vi "Sub_Conn_Status_FGV.vi"(6 "Connection Status in":T1=enum."Connection refused: not authorized", 8 "error in":errorcluster, 10 "Command":T2) -> (0 "error out":errorcluster, 4 "Connection Status out":T1=enum."Connection refused: not authorized")   [LabVIEW 2019, in "MQTT_Functions.lvlib"]
uses:
  MQTT_Functions.lvlib
  Controls/Connection_Return_Codes.ctl
  Controls/Conn_Stat_FGV_Cmds.ctl
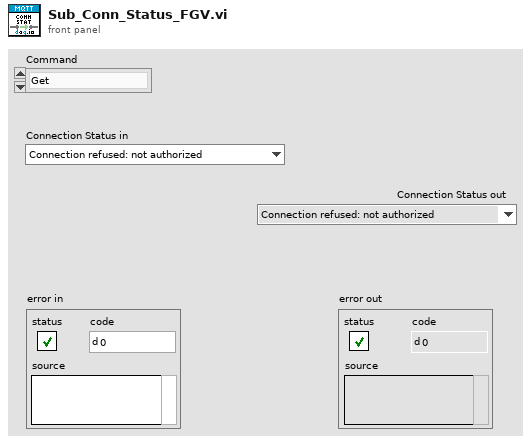
[diagram p1: front panel]
types:
  T1 = typedef "MQTT_Functions.lvlib/Connection_Return_Codes.ctl" = enum16{"Connection accepted", "Connection refused: unacceptable protocol version", "Connection refused: identifier rejected", "Connection refused: Server unavailable", "Connection refused: bad user name or password", "Connection refused: not authorized"}
  T2 = typedef "MQTT_Functions.lvlib/Conn_Stat_FGV_Cmds.ctl" = enum16{"Get", "Set"}
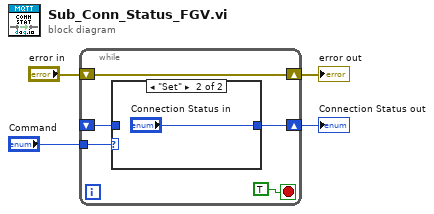
[diagram p0: block diagram]
diagram:
  n1 = while {
    shift-right: [w7] -> w3
    shift-left: _ -> [w6]
    tunnel: "Command" -> [w8]
    shift-right: [w5] -> w1
    shift-left: "error in" -> [w5]
    stop <- TRUE stop-if-true
    n2 = case shown="\"Set\"" w8 {
      tunnel: [w10 "Connection Status in"] -> w7
      tunnel: w6 -> [w10 _]
      frame "Get", Default {
      }
      frame "Set" {
      }
    }
  }
  "Connection Status out" <- w3
  "error out" <- w1
